vi "dB to Linear (scalar).vi"(1 "dB":dbl) -> (0 "linear":dbl)   [LabVIEW 2020]
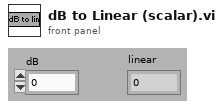
[diagram p1: front panel]
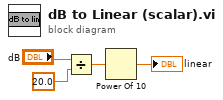
[diagram p0: block diagram]
diagram:
  n1 = Divide(x="dB", y=20.0) -> (x/y=w3:dbl)
  n2 = Power Of 10(x=w3) -> (10^x=→"linear":dbl)
